vi "manual_adjust.vi"(8 "error in":errorcluster, 11 "ConfigIn":T1={"SerialPort"="", "MinTime"=0.0, "baud rate"=9600, "data bits"=8, "parity"=enum."None", "stop bits"=10, "flow control"=0, "Steps"=0, "Active"=FALSE} {"flow control" items=["None", "XON/XOFF", "RTS/CTS", "XON/XOFF & RTS/CTS", "DTR/DSR", "XON/XOFF & DTR/DSR"]; "stop bits" items=["1.0"=10, "1.5"=15, "2.0"=20]; "data bits" min=5 max=8 step=1}) -> (0 "error out":errorcluster, 3 "ConfigOut":T1={"SerialPort"="", "MinTime"=0.0, "baud rate"=9600, "data bits"=8, "parity"=enum."None", "stop bits"=10, "flow control"=0, "Steps"=0, "Active"=FALSE} {"flow control" items=["None", "XON/XOFF", "RTS/CTS", "XON/XOFF & RTS/CTS", "DTR/DSR", "XON/XOFF & DTR/DSR"]; "stop bits" items=["1.0"=10, "1.5"=15, "2.0"=20]; "data bits" min=5 max=8 step=1})   [LabVIEW 2016]
uses:
  step_motor_data.ctl
panel:
  out "Passos":i32
  in  "OK":bool
  in  "UnitStep":bool
  # "Ajuste manual do avanço\nIncrementar: um passo do motor\nFinalizar: continuar ensaio"
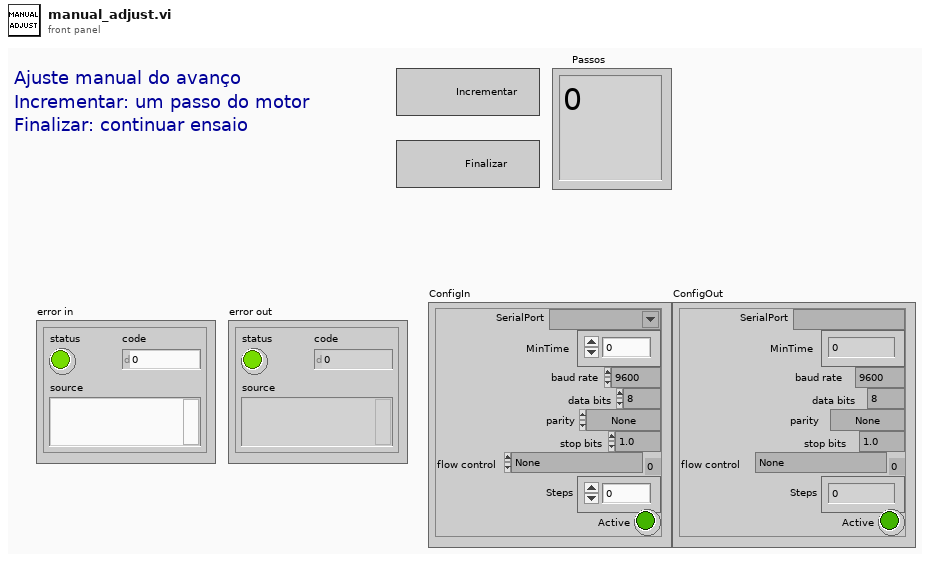
[diagram p1: front panel]
types:
  T1 = typedef "step_motor_data.ctl" = cluster{"SerialPort":refnum<visa-resource-name>, "MinTime":dbl, "baud rate":u32, "data bits":u16, "parity":enum16{"None", "Odd", "Even", "Mark", "Space"}, "stop bits":u16, "flow control":u16, "Steps":i32, "Active":bool}
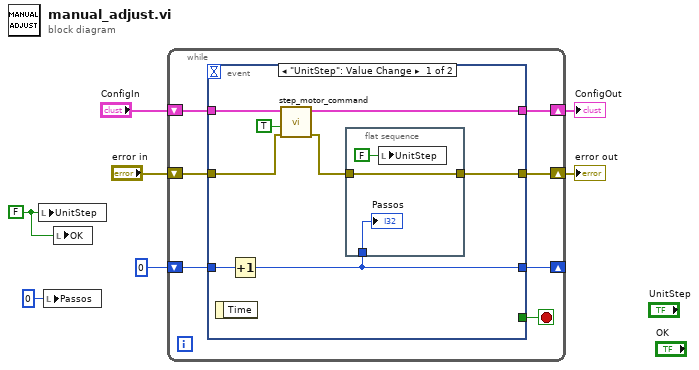
[diagram p0: block diagram]
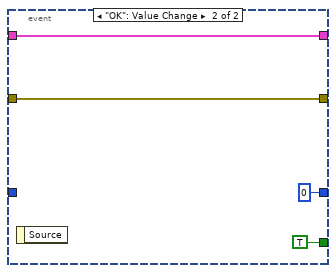
[diagram p2: hidden frame]
diagram:
  w3 = FALSE ("UnitStep")
  n1 = local write "UnitStep"(w3) -> ()
  n2 = local write "Passos"(0 ("Passos")) -> ()
  n3 = local write "OK"(w3) -> ()
  n4 = while {
    shift-right: [w13] -> w2
    shift-left: "ConfigIn" -> [w14]
    shift-right: [w11] -> w4
    shift-left: "error in" -> [w12]
    shift-right: [w10] -> _
    shift-left: 0 -> [w9]
    stop <- w8 stop-if-true
    n5 = event shown="[0] \"UnitStep\": Value Change" {
      selector: _ -> [_ _]
      dyn-events: _ -> [_ _]
      timeout: _ -> [_ _]
      tunnel: w14 -> [w21 w27]
      tunnel: [w20 w27] -> w13
      tunnel: w12 -> [w19 w28]
      tunnel: [w16 w28] -> w11
      tunnel: [w15 0] -> w10
      tunnel: w9 -> [w18 _]
      tunnel: [_ TRUE ("UnitStep")] -> w8
      event "UnitStep": Value Change {
        n6 = event-data() -> ()  [unwired: 1 in, 1 out]
        n7 = Increment(x=w18) -> (x+1=w15:i32)
        n8 = call "step_motor_command.vi"("error in"=w19, "Ajuste?"=TRUE, "step_motor_data"=w21) -> ("error out"=w17:errorcluster, "output cluster"=w20:T1)  [unwired: 6 in, 1 out]
        n9 = flat-sequence {
          tunnel: w17 -> [w25]
          tunnel: [w25] -> w16
          tunnel: w15 -> [w24]
          frame #0 {
            n10 = local write "UnitStep"(FALSE ("UnitStep")) -> ()
            "Passos" <- w24
          }
        }
      }
      event "OK": Value Change {
        n11 = event-data() -> ()  [unwired: 1 in, 1 out]
      }
    }
  }
  "error out" <- w4
  "ConfigOut" <- w2
